vi "Logfile_Data_Header.vi"(2 "System Monitor Cluster":T1={"Time"=[], "LI1CH1"=[], "LI1CH2"=[], "LI2CH1"=[], "LI2CH2"=[], "LI3CH1"=[], "LI3CH2"=[], "Field"=[], "Temperature"=[], "Temperature 2"=[], "Temperatrue 3"=[], "Nitrogen_Level"=[], "Helium_Level"=[], "Heater_LS370"=[], "Sorb_Heater"=[], "Still_Heater"=[], "Capacity"=[], "Loss"=[], "Magnet_Temperature"=[], "Lambda_Pressure"=[], "Lambda_Needle_Valve"=[], "LS370-CH1-T"=[], "LS370-CH2-T"=[], "LS370-CH3-T"=[], "LS370-CH4-T"=[], "LS370-TC-T"=[], "LS370-CH1-R"=[], "LS370-CH2-R"=[], "LS370-CH3-R"=[], "LS370-CH4-R"=[], "LS370-TC-R"=[], "LS372-CH1-T"=[], "LS372-CH2-T"=[], "LS372-CH3-T"=[], "LS372-CH4-T"=[], "LS372-CH5-T"=[], "LS372-CH1-R"=[], "LS372-CH2-R"=[], "LS372-CH3-R"=[], "LS372-CH4-R"=[], "LS372-CH5-R"=[], "Nada"=[nan], "Keithley_Res"=[], "Keithley_Current"=[], "VTI_Heater"=[], "VTI_Needle Valve"=[], "LS340_Heater"=[], "Keithley_6221_Amplitude"=[], "Keithley_6221_Frequency"=[], "Condense_Pressure"=[], "Still_Pressure"=[], "FP_Out_Pressure"=[], "Dump_Pressure"=[], "V1"=[], "V2"=[], "V4"=[], "V5"=[], "V9"=[], "Forepump"=[], "Compressor"=[], "Keihtley_6221_Offset"=[], "BoxTemp"=[], "By"=[], "Bz"=[], "Phi"=[]}) -> (0 "Data Line":string)   [LabVIEW 2016]
uses:
  Global/Global Variables/System Monitor Cluster.ctl
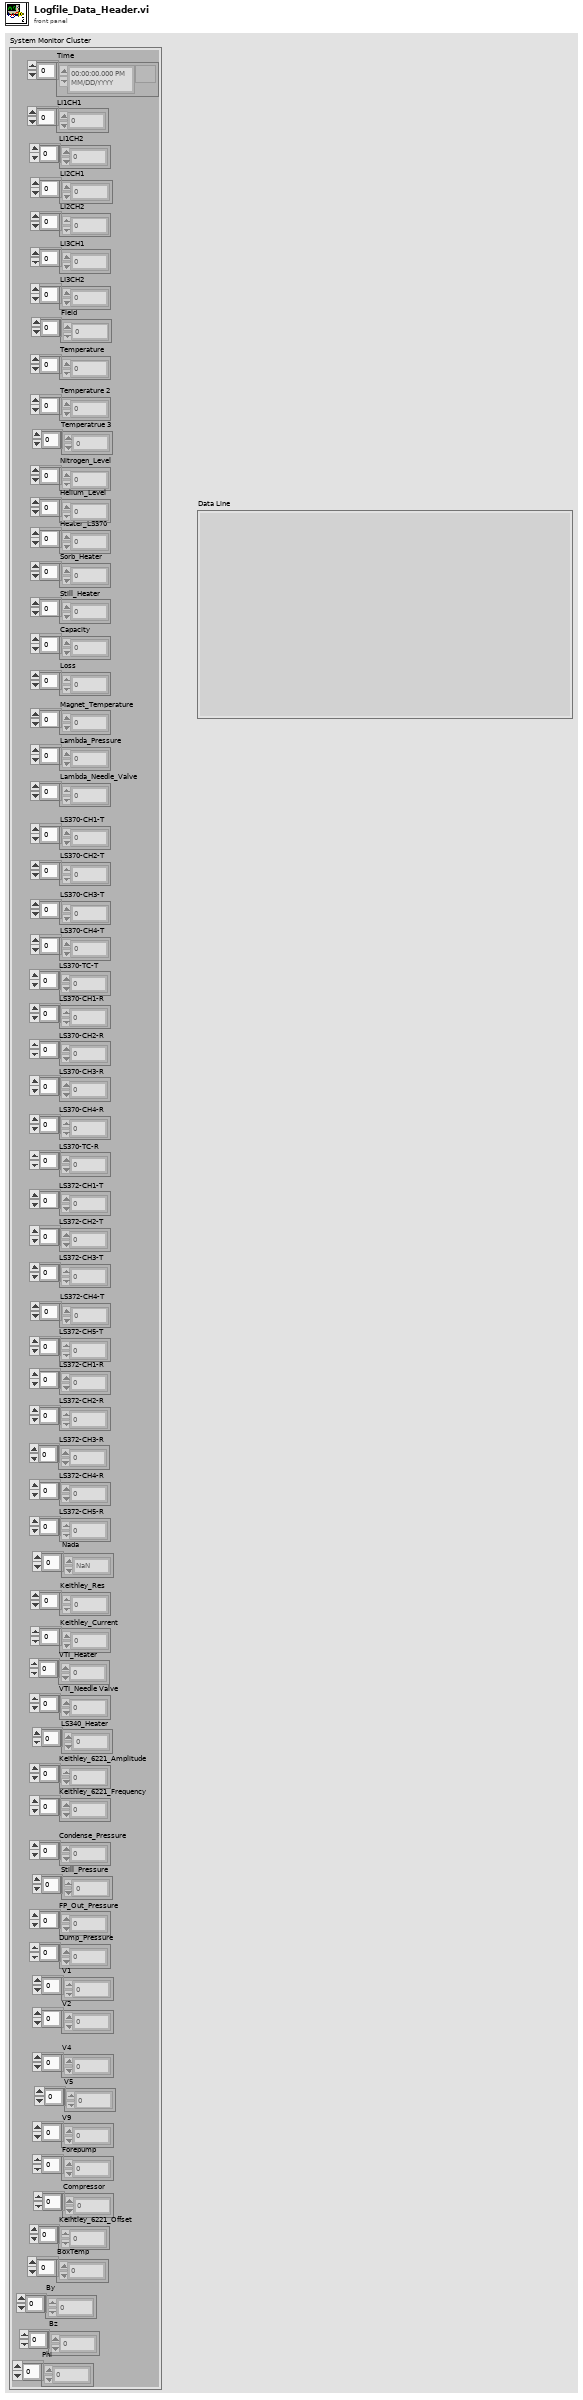
[diagram p1: front panel]
types:
  T1 = typedef "System Monitor Cluster.ctl" = cluster{"Time":timestamp[], "LI1CH1":dbl[], "LI1CH2":dbl[], "LI2CH1":dbl[], "LI2CH2":dbl[], "LI3CH1":dbl[], "LI3CH2":dbl[], "Field":dbl[], "Temperature":dbl[], "Temperature 2":dbl[], "Temperatrue 3":dbl[], "Nitrogen_Level":dbl[], "Helium_Level":dbl[], "Heater_LS370":dbl[], "Sorb_Heater":dbl[], "Still_Heater":dbl[], "Capacity":dbl[], "Loss":dbl[], "Magnet_Temperature":dbl[], "Lambda_Pressure":dbl[], "Lambda_Needle_Valve":dbl[], "LS370-CH1-T":dbl[], "LS370-CH2-T":dbl[], "LS370-CH3-T":dbl[], "LS370-CH4-T":dbl[], "LS370-TC-T":dbl[], "LS370-CH1-R":dbl[], "LS370-CH2-R":dbl[], "LS370-CH3-R":dbl[], "LS370-CH4-R":dbl[], "LS370-TC-R":dbl[], "LS372-CH1-T":dbl[], "LS372-CH2-T":dbl[], "LS372-CH3-T":dbl[], "LS372-CH4-T":dbl[], "LS372-CH5-T":dbl[], "LS372-CH1-R":dbl[], "LS372-CH2-R":dbl[], "LS372-CH3-R":dbl[], "LS372-CH4-R":dbl[], "LS372-CH5-R":dbl[], "Nada":dbl[], "Keithley_Res":dbl[], "Keithley_Current":dbl[], "VTI_Heater":dbl[], "VTI_Needle Valve":dbl[], "LS340_Heater":dbl[], "Keithley_6221_Amplitude":dbl[], "Keithley_6221_Frequency":dbl[], "Condense_Pressure":dbl[], "Still_Pressure":dbl[], "FP_Out_Pressure":dbl[], "Dump_Pressure":dbl[], "V1":dbl[], "V2":dbl[], "V4":dbl[], "V5":dbl[], "V9":dbl[], "Forepump":dbl[], "Compressor":dbl[], "Keihtley_6221_Offset":dbl[], "BoxTemp":dbl[], "By":dbl[], "Bz":dbl[], "Phi":dbl[]}
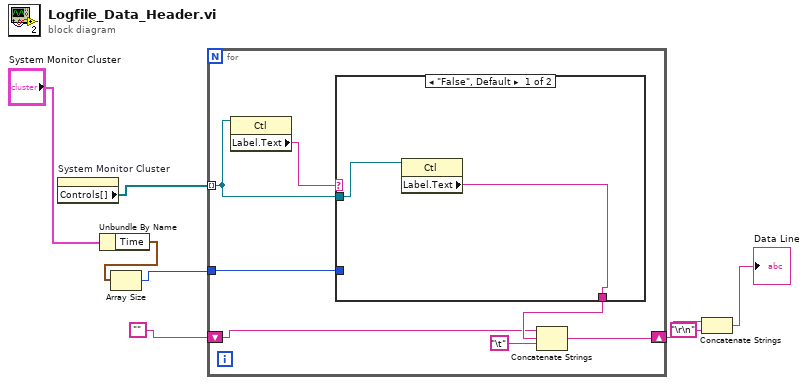
[diagram p0: block diagram]
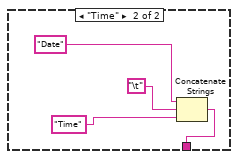
[diagram p2: hidden frame]
diagram:
  n1 = property on="System Monitor Cluster" class="Clust (strict)"() -> ("Controls[]"=w8:refnum<vi>[])  [unwired: 2 in, 2 out]
  n2 = Unbundle By Name("System Monitor Cluster") -> ("Time"=w2:timestamp[])
  n3 = Array Size(array=w2) -> (size(s)=w1:i32)
  n4 = for {
    tunnel: w8 -> [w15] mode=indexing
    shift-right: [w10] -> w6
    shift-left: "" -> [w11]
    tunnel: w1 -> [w9]
    n5 = property class="Ctl"(reference=w15) -> ("Label.Text"=w14:string)  [unwired: 1 in, 2 out]
    n6 = case shown="\"False\", Default" w14 {
      tunnel: w15 -> [w17 _]
      tunnel: [w16 w21] -> w13
      tunnel: w9 -> [_ _]
      frame "False", Default {
        n7 = property class="Ctl"(reference=w17) -> ("Label.Text"=w16:string)  [unwired: 1 in, 2 out]
      }
      frame "Time" {
        n8 = Concatenate Strings("Date", "\t", "Time") -> (w21:string)
      }
    }
    n9 = Concatenate Strings(w11, w13, "\t") -> (w10:string)
  }
  n10 = Concatenate Strings(w6, "\r\n") -> (→"Data Line":string)
